vi "Ramp Trans Up.vi"(9 "Time (ms)":u32=500, 11 "VI Ref In":refnum<vi>) -> ()   [LabVIEW 2016, in "Rectangle Mask.lvclass"]
uses:
  Classes/Rectangle Mask/Rectangle Mask.lvclass
panel:
  out "VI Ref Out":refnum<vi>
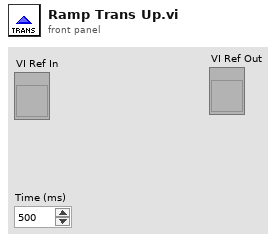
[diagram p1: front panel]
types:
  T1 = enum32{"Invalid", "Standard", "Closed", "Hidden", "Minimized", "Maximized"}
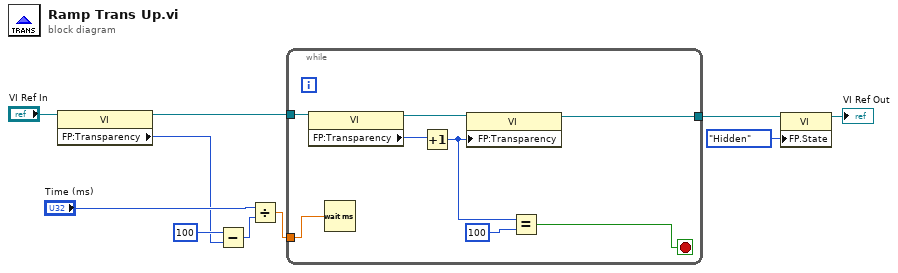
[diagram p0: block diagram]
diagram:
  n1 = property class="VI"(reference="VI Ref In") -> (reference out=w4:refnum<vi>, "FP:Transparency"=w3:u8)  [unwired: 1 in, 1 out]
  n2 = Subtract(x=u32 100, y=w3) -> (x-y=w8:u32)
  n3 = Divide(x="Time (ms)", y=w8) -> (x/y=w10:dbl)
  n4 = while {
    tunnel: w10 -> [w18]
    tunnel: w4 -> [w17]
    tunnel: [w12] -> w6
    stop <- w13 stop-if-true
    n5 = property class="VI"(reference=w17) -> (reference out=w15:refnum<vi>, "FP:Transparency"=w16:u8)  [unwired: 1 in, 1 out]
    n6 = Wait (ms)(milliseconds to wait=w18) -> ()  [unwired: 1 out]
    n7 = Increment(x=w16) -> (x+1=w14:u8)
    n8 = property class="VI"(reference=w15, "FP:Transparency"=w14) -> (reference out=w12:refnum<vi>)  [unwired: 1 in, 1 out]
    n9 = Equal?(x=w14, y=u8 100) -> (x = y?=w13:bool)
  }
  n10 = property class="VI"(reference=w6, "FP.State"=T1."Hidden" ("Front Panel Window:State")) -> (reference out=→"VI Ref Out":refnum<vi>)  [unwired: 1 in, 1 out]
